vi "Parse String.vi"(8 "error in (no error)":errorcluster, 10 "Index In":i32, 11 "JSON String":string) -> (0 "error out":errorcluster, 1 "Parsed String":string, 2 "Index Out":i32, 3 "JSON Value out":refnum<class "JSON Value.lvclass">)   [LabVIEW 2016, in "JSON Value.lvclass"]
uses:
  JSON Value.lvclass
  subVIs/Errors.ctl
  New JSON Value/New JSON (String).vi
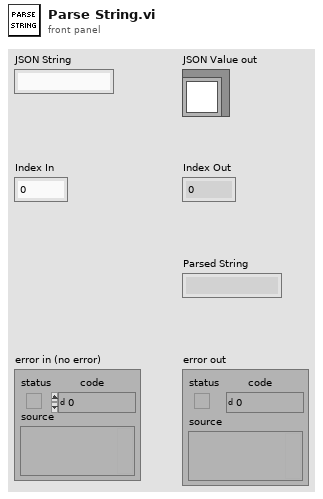
[diagram p1: front panel]
types:
  T1 = typedef "JSON Value.lvclass/Errors.ctl" = enum8{"No key", "Key path type", "Array OOB", "Type Mismatch", "Invalid Token"}
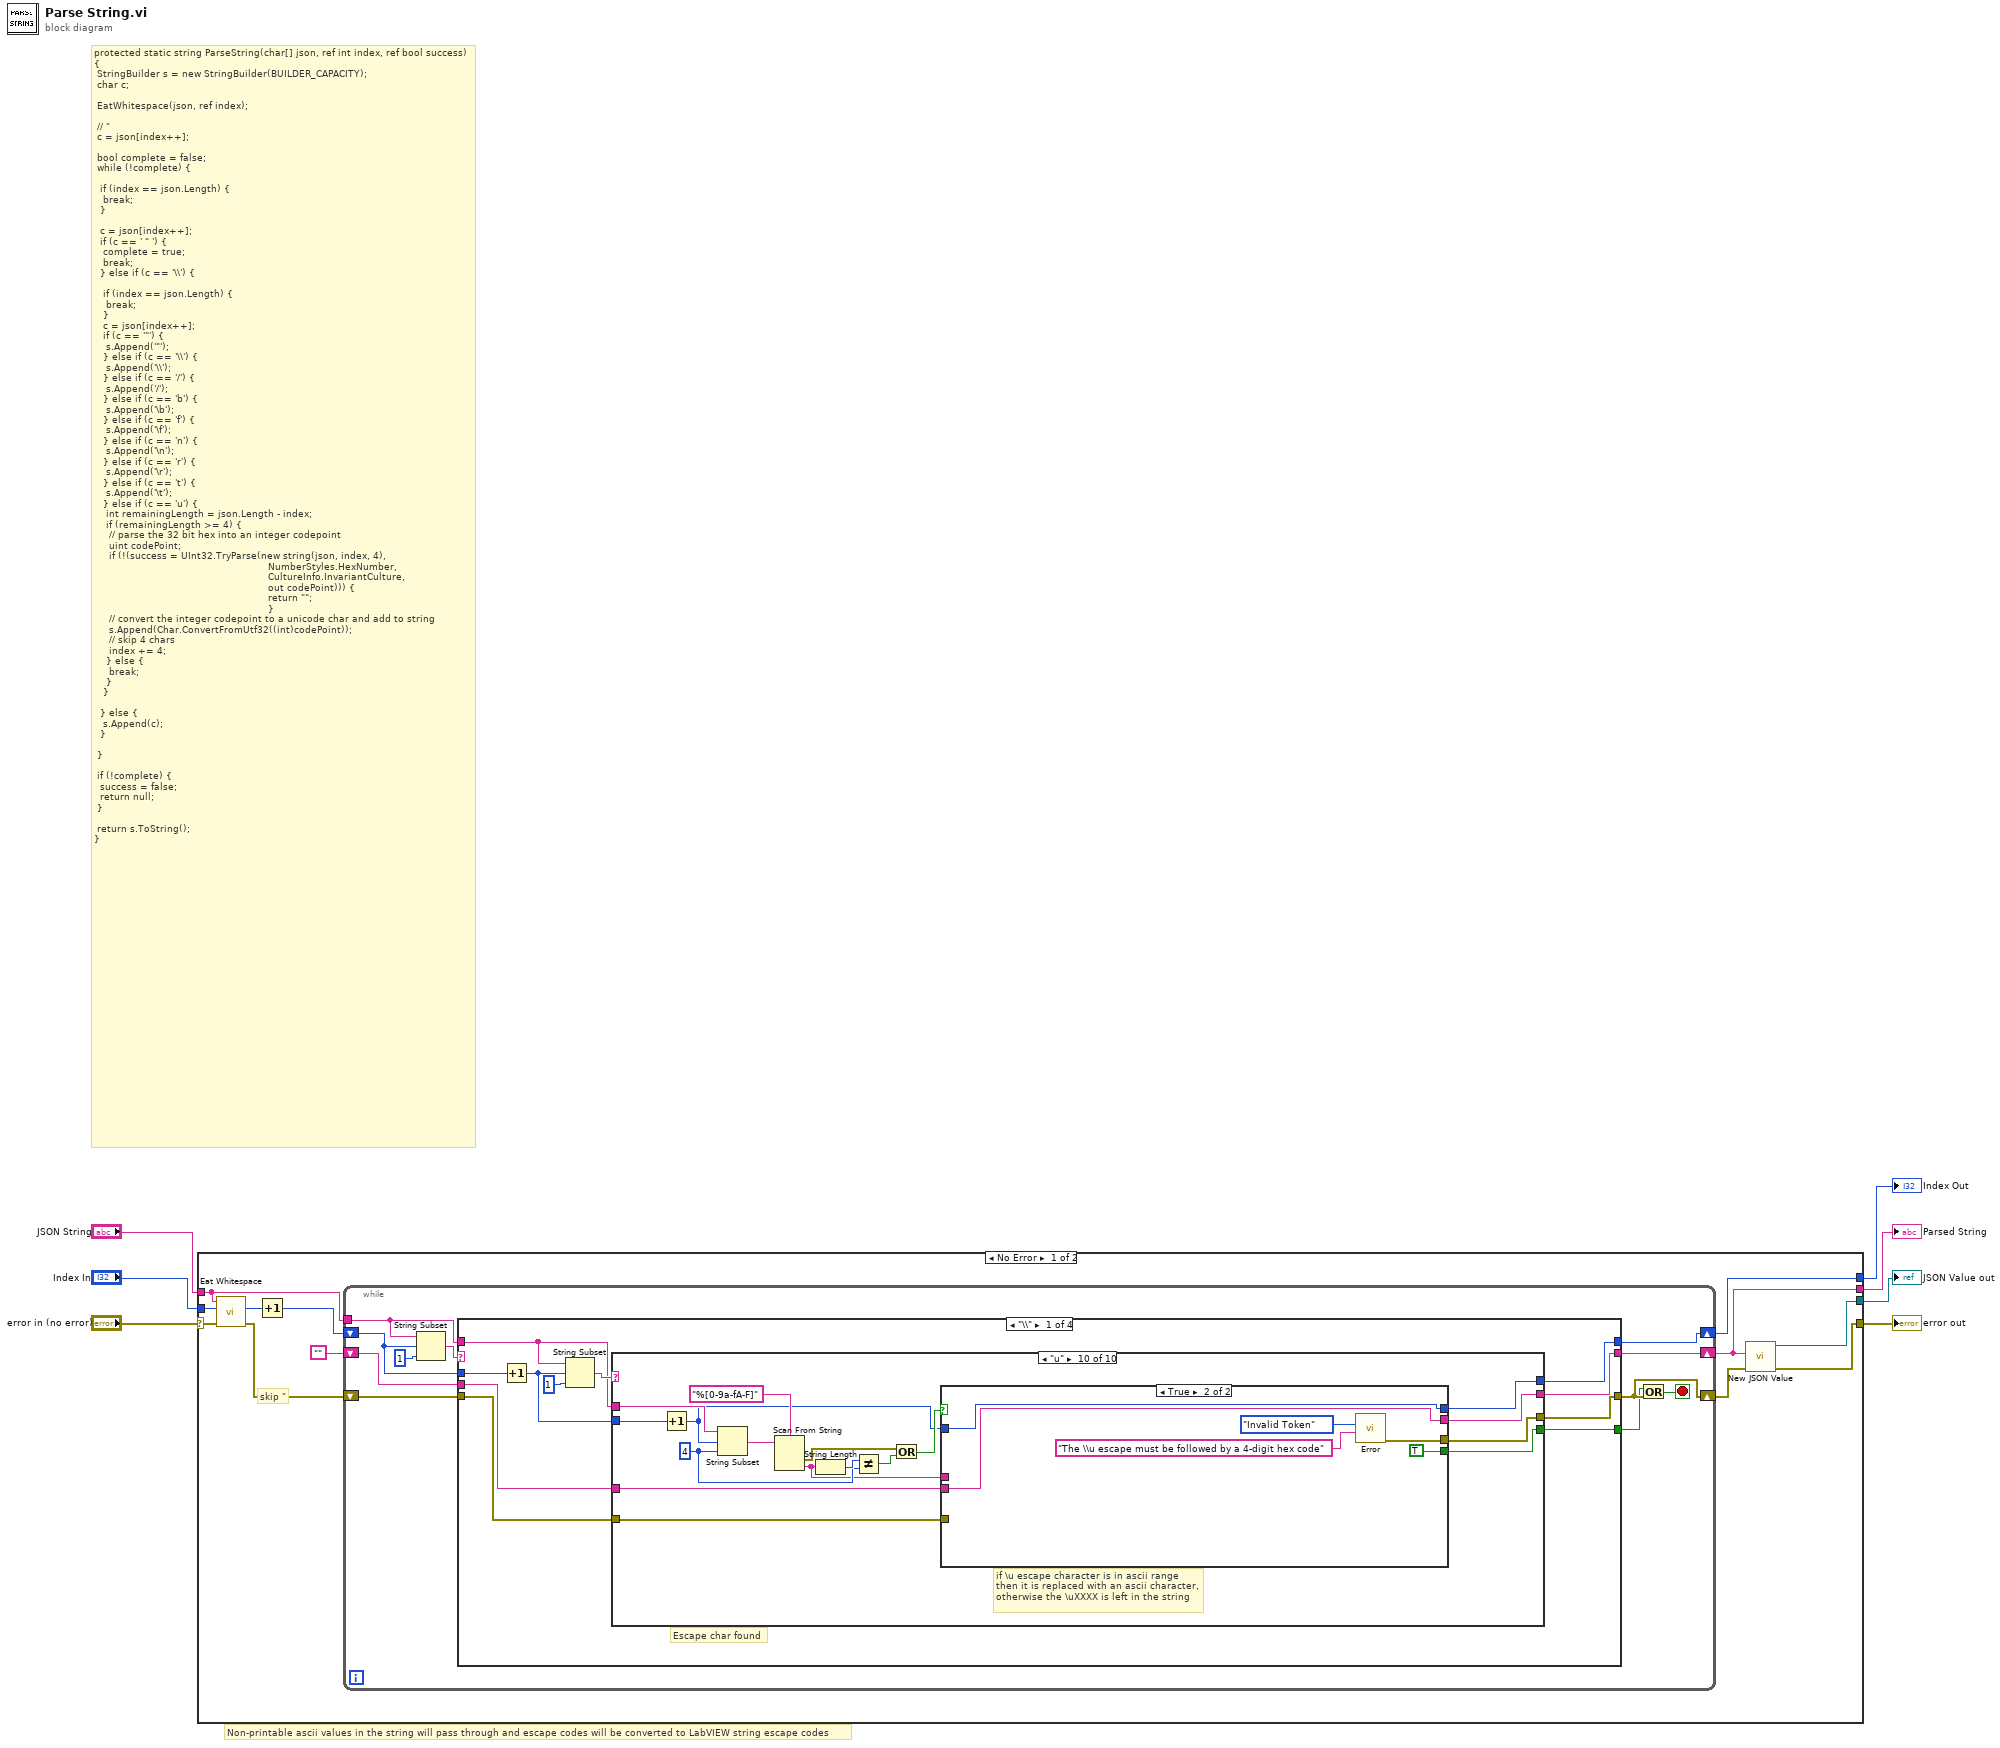
[diagram p0: block diagram]
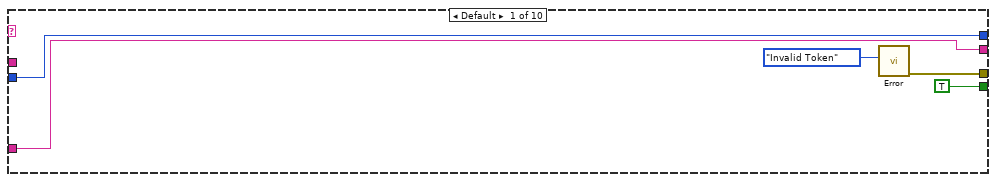
[diagram p2: hidden frame]
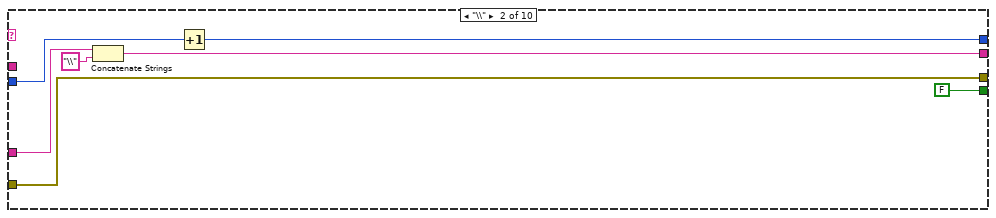
[diagram p3: hidden frame]
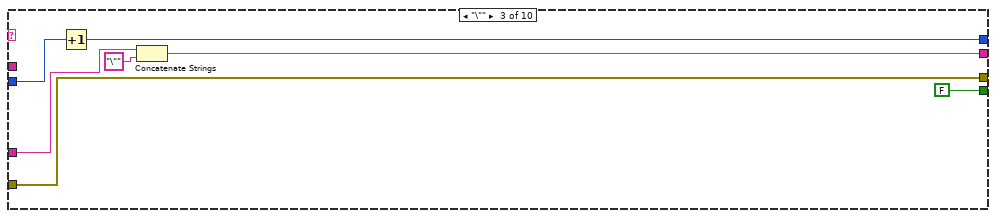
[diagram p4: hidden frame]
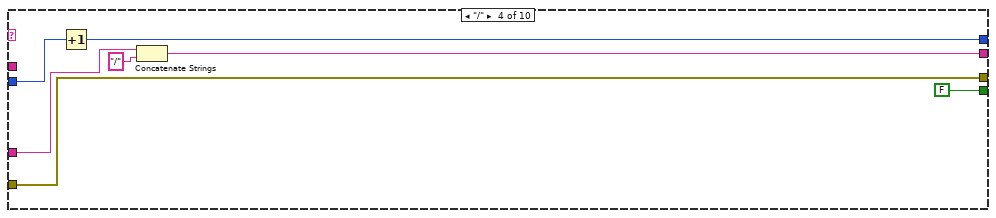
[diagram p5: hidden frame]
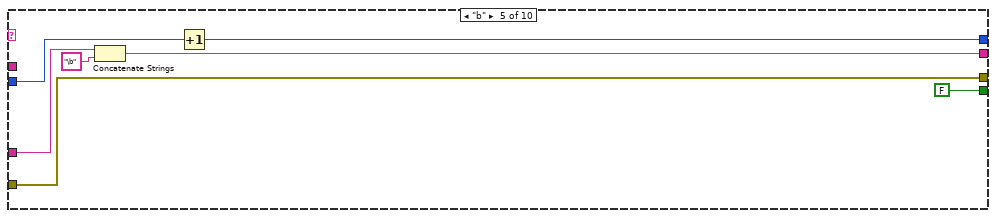
[diagram p6: hidden frame]
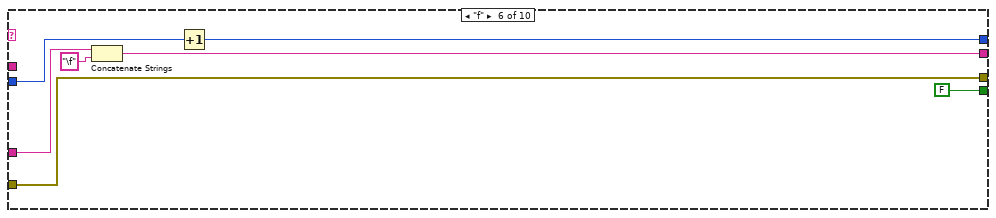
[diagram p7: hidden frame]
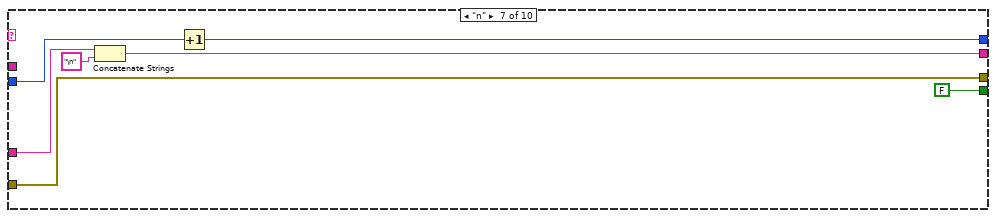
[diagram p8: hidden frame]
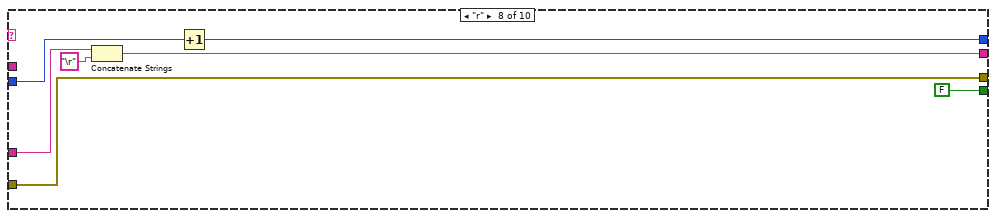
[diagram p9: hidden frame]
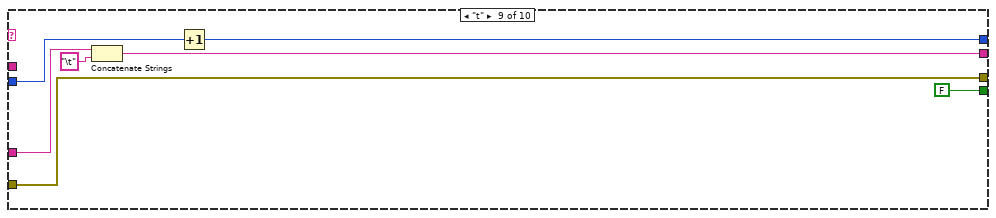
[diagram p10: hidden frame]
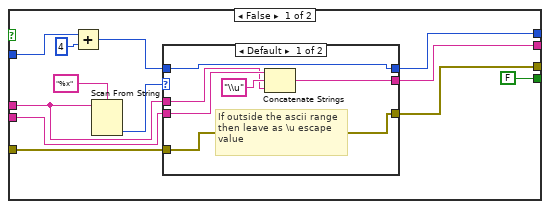
[diagram p11: hidden frame]
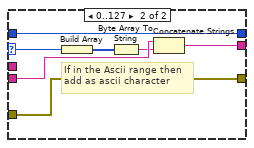
[diagram p12: hidden frame]
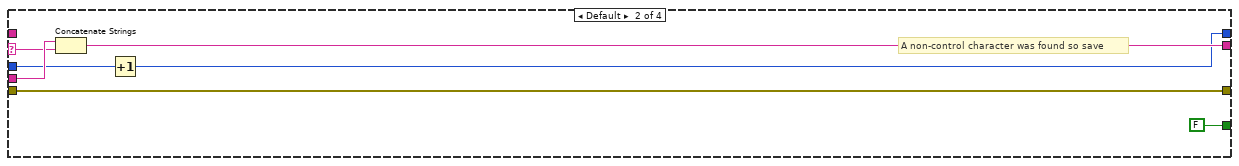
[diagram p13: hidden frame]
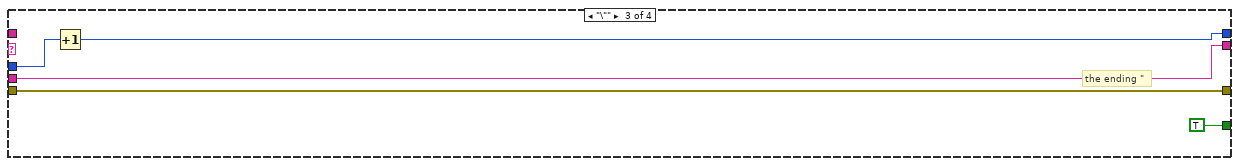
[diagram p14: hidden frame]
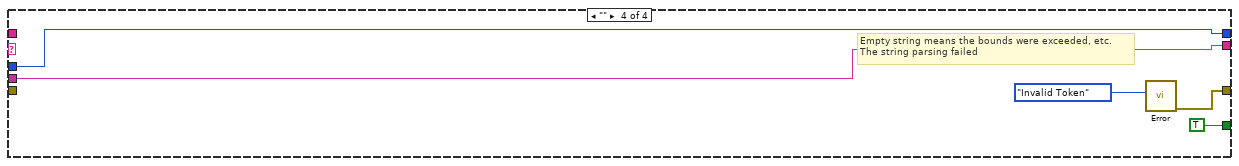
[diagram p15: hidden frame]
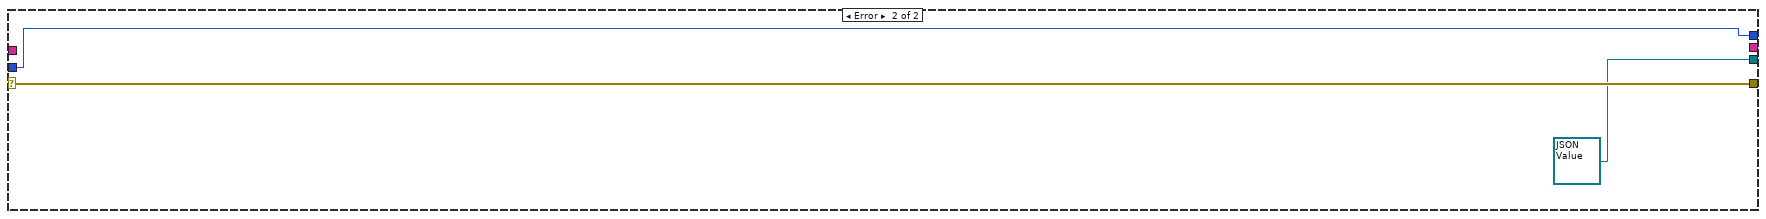
[diagram p16: hidden frame]
diagram:
  # "Non-printable ascii values in the string will pass through and escape codes will be converted to LabVIEW string escape codes"
  # "protected static string ParseString(char[] json, ref int index, ref bool success)\n{\n\tStringBuilder s = new StringBuilder(BUILDER_CAPACITY);\n\tchar c;\n\n\tEatWhitespace(json, ref index);\n\n\t// \"\n\tc = json[index++];\n\n\tbool complete = false;\n\twhile (!complete) {\n\n\t\tif (index == json.Length) {\n\t\t\tbreak;\n\t\t}\n\n\t\tc = json[index++];\n\t\tif (c == ' \" ') {\n\t\t\tcomplete = true;\n\t\t\tbreak;\n\t\t} else if (c == '\\\\') {\n\n\t\t\tif (index == json.Length) {\n\t\t\t\tbreak;\n\t\t\t}\n\t\t\tc = json[index++];\n\t\t\tif (c == '\"') {\n\t\t\t\ts.Append('\"');\n\t\t\t} else if (c == '\\\\') {\n\t\t\t\ts.Append('\\\\');\n\t\t\t} else if (c == '/') {\n\t\t\t\ts.Append('/');\n\t\t\t} else if (c == 'b') {\n\t\t\t\ts.Append('\\b');\n\t\t\t} else if (c == 'f') {\n\t\t\t\ts.Append('\\f');\n\t\t\t} else if (c == 'n') {\n\t\t\t\ts.Append('\\n');\n\t\t\t} else if (c == 'r') {\n\t\t\t\ts.Append('\\r');\n\t\t\t} else if (c == 't') {\n\t\t\t\ts.Append('\\t');\n\t\t\t} else if (c == 'u') {\n\t\t\t\tint remainingLength = json.Length - index;\n\t\t\t\tif (remainingLength >= 4) {\n\t\t\t\t\t// parse the 32 bit hex into an integer codepoint\n\t\t\t\t\tuint codePoint;\n\t\t\t\t\tif (!(success = UInt32.TryParse(new string(json, index, 4),\n                                                          NumberStyles.HexNumber,\n                                                          CultureInfo.InvariantCulture,\n                                                          out codePoint))) {\n\t\t\t\t\t\t                                                    return \"\";\n\t\t\t\t\t                                                     }\n\t\t\t\t\t// convert the integer codepoint to a unicode char and add to string\n\t\t\t\t\ts.Append(Char.ConvertFromUtf32((int)codePoint));\n\t\t\t\t\t// skip 4 chars\n\t\t\t\t\tindex += 4;\n\t\t\t\t} else {\n\t\t\t\t\tbreak;\n\t\t\t\t}\n\t\t\t}\n\n\t\t} else {\n\t\t\ts.Append(c);\n\t\t}\n\n\t}\n\n\tif (!complete) {\n\t\tsuccess = false;\n\t\treturn null;\n\t}\n\n\treturn s.ToString();\n}"
  n1 = case shown="No Error" "error in (no error)" {
    selector: "error in (no error)" -> [w19 w169]
    tunnel: [w11 w169] -> w6
    tunnel: "Index In" -> [w14 w170]
    tunnel: [w13 w170] -> w4
    tunnel: [w10 refnum<class "JSON Value.lvclass"> refnum ("JSON out")] -> w3
    tunnel: [w8 _] -> w2
    tunnel: "JSON String" -> [w9 _]
    frame No Error {
      # "skip \""
      n2 = call "Eat Whitespace.vi"("error in (no error)"=w19, "Index In"=w14, "JSON String"=w9) -> ("error out"=w15:errorcluster, "Index Out"=w18:i32)  [unwired: 7 in]
      n3 = Increment(x=w18) -> (x+1=w17:i32)
      n4 = while {
        tunnel: w9 -> [w26]
        shift-right: [w27] -> w8
        shift-left: "" -> [w28]
        shift-right: [w23] -> w13
        shift-left: w17 -> [w24]
        shift-right: [w22] -> w12
        shift-left: w15 -> [w25]
        stop <- w20 stop-if-true
        n5 = String Subset(string=w26, offset (0)=w24, length (rest)=1 ("length (rest)")) -> (substring=w29:string)
        n6 = case shown="\"\\\\\"" w29 {
          selector: w29 -> [_ w156 _ _]
          tunnel: [w32 FALSE TRUE TRUE] -> w21
          tunnel: w28 -> [w38 w157 w161 w167]
          tunnel: [w37 w155 w161 w167] -> w27
          tunnel: w24 -> [w41 w154 w160 w165]
          tunnel: w26 -> [w31 _ _ _]
          tunnel: [w36 w153 w159 w165] -> w23
          tunnel: w25 -> [w34 w151 w158 _]
          tunnel: [w33 w151 w158 w164] -> w22
          frame "\\" {
            # "Escape char found"
            n7 = Increment(x=w41) -> (x+1=w35:i32)
            n8 = String Subset(string=w31, offset (0)=w35, length (rest)=1 ("length (rest)")) -> (substring=w39:string)
            n9 = case shown="\"u\"" w39 {
              tunnel: w38 -> [w45 w53 w60 w67 w74 w81 w88 w95 w102 w110]
              tunnel: [w45 w52 w59 w66 w73 w80 w87 w94 w101 w106] -> w37
              tunnel: [w44 w49 w56 w63 w70 w77 w84 w91 w98 w104] -> w36
              tunnel: w35 -> [w44 w50 w57 w64 w71 w78 w85 w92 w99 w118]
              tunnel: w34 -> [_ w48 w55 w62 w69 w76 w83 w90 w97 w109]
              tunnel: [w43 w48 w55 w62 w69 w76 w83 w90 w97 w108] -> w33
              tunnel: [TRUE FALSE FALSE FALSE FALSE FALSE FALSE FALSE FALSE w107] -> w32
              tunnel: w31 -> [_ _ _ _ _ _ _ _ _ w119]
              frame Default {
                n10 = call "Error.vi"("Error"=Errors."Invalid Token") -> ("error out"=w43:errorcluster)  [unwired: 9 in]
              }
              frame "\\" {
                n11 = Concatenate Strings(w53, "\\" ("string")) -> (w52:string)
                n12 = Increment(x=w50) -> (x+1=w49:i32)
              }
              frame "\"" {
                n13 = Increment(x=w57) -> (x+1=w56:i32)
                n14 = Concatenate Strings(w60, "\"" ("string")) -> (w59:string)
              }
              frame "/" {
                n15 = Increment(x=w64) -> (x+1=w63:i32)
                n16 = Concatenate Strings(w67, "/" ("string")) -> (w66:string)
              }
              frame "b" {
                n17 = Concatenate Strings(w74, "\b" ("string")) -> (w73:string)
                n18 = Increment(x=w71) -> (x+1=w70:i32)
              }
              frame "f" {
                n19 = Concatenate Strings(w81, "\f" ("string")) -> (w80:string)
                n20 = Increment(x=w78) -> (x+1=w77:i32)
              }
              frame "n" {
                n21 = Concatenate Strings(w88, "\n" ("string")) -> (w87:string)
                n22 = Increment(x=w85) -> (x+1=w84:i32)
              }
              frame "r" {
                n23 = Concatenate Strings(w95, "\r" ("string")) -> (w94:string)
                n24 = Increment(x=w92) -> (x+1=w91:i32)
              }
              frame "t" {
                n25 = Concatenate Strings(w102, "\t" ("string")) -> (w101:string)
                n26 = Increment(x=w99) -> (x+1=w98:i32)
              }
              frame "u" {
                w112 = 4 ("length (rest)")
                # "if \\u escape character is in ascii range\nthen it is replaced with an ascii character,\notherwise the \\uXXXX is left in the string"
                n27 = Increment(x=w118) -> (x+1=w105:i32)
                n28 = String Subset(string=w119, offset (0)=w105, length (rest)=w112) -> (substring=w117:string)
                n29 = Scan From String(format string="%[0-9a-fA-F]", input string=w117) -> (error out=w113:errorcluster, output 1=w103:string)  [unwired: 3 in, 2 out]
                n30 = String Length(string=w103) -> (length=w115:i32)
                n31 = Not Equal?(x=w115, y=w112) -> (x != y?=w114:bool)
                n32 = Or(x=w113, y=w114) -> (x .or. y?=w111:bool)
                n33 = case shown="True" w111 {
                  tunnel: w110 -> [w128 w149]
                  tunnel: w109 -> [w126 _]
                  tunnel: [w125 w145] -> w108
                  tunnel: [FALSE TRUE] -> w107
                  tunnel: [w127 w149] -> w106
                  tunnel: w105 -> [w121 w148]
                  tunnel: [w124 w148] -> w104
                  tunnel: w103 -> [w123 _]
                  frame False {
                    n34 = Add(x=w121, y=4) -> (x+y=w120:i32)
                    n35 = Scan From String(format string="%x", input string=w123) -> (output 1=w129:u32)  [unwired: 3 in, 3 out]
                    n36 = case shown="Default" w129 {
                      selector: w129 -> [_ w144]
                      tunnel: w128 -> [w134 w142]
                      tunnel: [w135 w141] -> w127
                      tunnel: w126 -> [w136 w140]
                      tunnel: [w136 w140] -> w125
                      tunnel: [w137 w138] -> w124
                      tunnel: w123 -> [w132 _]
                      tunnel: w120 -> [w137 w138]
                      frame Default {
                        # "If outside the ascii range\nthen leave as \\u escape\nvalue"
                        n37 = Concatenate Strings(w134, "\\u" ("string"), w132) -> (w135:string)
                      }
                      frame 0..127 {
                        # "If in the Ascii range then\nadd as ascii character"
                        n38 = Build Array(w144) -> (w143:u32[])
                        n39 = Byte Array To String(unsigned byte array=w143) -> (string=w139:string)
                        n40 = Concatenate Strings(w142, w139) -> (w141:string)
                      }
                    }
                  }
                  frame True {
                    n41 = call "Error.vi"("Data"="The \\u escape must be followed by a 4-digit hex code" ("source"), "Error"=Errors."Invalid Token") -> ("error out"=w145:errorcluster)  [unwired: 8 in]
                  }
                }
              }
            }
          }
          frame Default {
            # "A non-control character was found so save"
            n42 = Concatenate Strings(w157, w156) -> (w155:string)
            n43 = Increment(x=w154) -> (x+1=w153:i32)
          }
          frame "\"" {
            # "the ending \""
            n44 = Increment(x=w160) -> (x+1=w159:i32)
          }
          frame "" {
            # "Empty string means the bounds were exceeded, etc.\nThe string parsing failed"
            n45 = call "Error.vi"("Error"=Errors."Invalid Token") -> ("error out"=w164:errorcluster)  [unwired: 9 in]
          }
        }
        n46 = Or(x=w21, y=w22) -> (x .or. y?=w20:bool)
      }
      n47 = call-poly "New JSON Value.vi"("error in (no error)"=w12, "value"=w8) -> ("error out"=w11:errorcluster, "JSON Value out"=w10:refnum<class "JSON Value.lvclass">)  [unwired: 8 in]
    }
    frame Error {
    }
  }
  "error out" <- w6
  "Index Out" <- w4
  "JSON Value out" <- w3
  "Parsed String" <- w2
